vi "BuildUpdateQuery.vi"(8 "error in (no error)":errorcluster, 10 "QueryBuilderData":T1) -> (0 "error out":errorcluster, 2 "Query":string)   [LabVIEW 2022 SP3]
uses:
  DataTypes/QuiryBuilderData--Cluster.ctl
  <vilib>/Utility/error.llb/Trim Whitespace One-Sided.vi
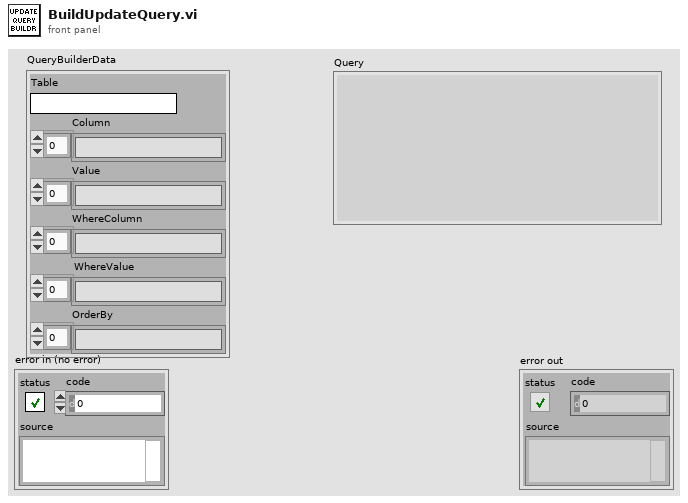
[diagram p1: front panel]
types:
  T1 = typedef "QuiryBuilderData--Cluster.ctl" = cluster{"Table":string, "Column":string[], "Value":string[], "WhereColumn":string[], "WhereValue":string[], "OrderBy":string[]}
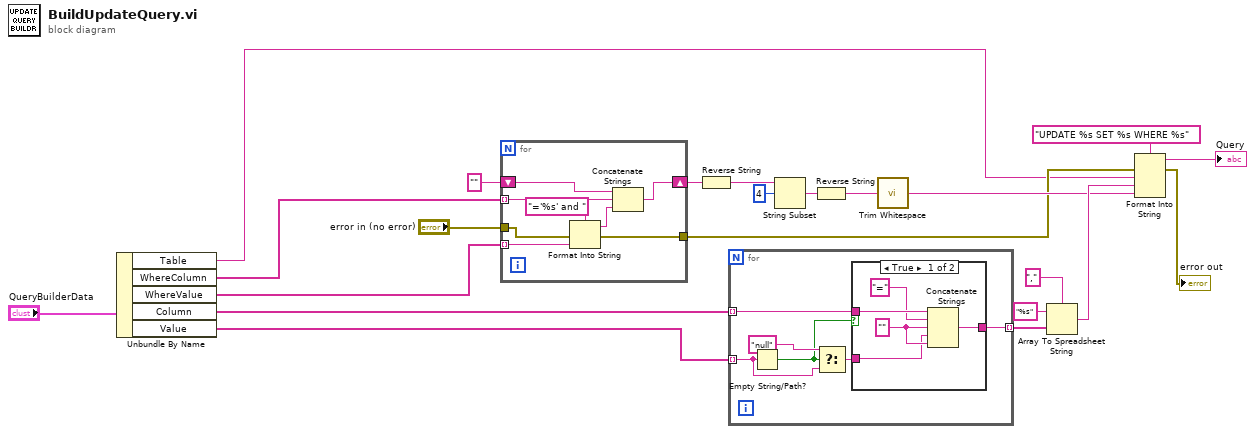
[diagram p0: block diagram]
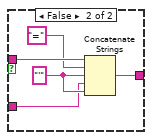
[diagram p2: hidden frame]
diagram:
  n1 = Unbundle By Name("QueryBuilderData") -> ("Table"=w2:string, "WhereColumn"=w3:string[], "WhereValue"=w4:string[], "Column"=w6:string[], "Value"=w5:string[])
  n2 = for {
    tunnel: w3 -> [w30] mode=indexing
    shift-right: [w29] -> w16
    shift-left: "" -> [w28]
    tunnel: w4 -> [w25] mode=indexing
    tunnel: "error in (no error)" -> [w24]
    tunnel: [w23] -> w9
    n3 = Format Into String(format string="='%s' and " ("string"), error in=w24, w25) -> (resulting string=w26:string, error out=w23:errorcluster)  [unwired: 1 in]
    n4 = Concatenate Strings(w28, w30, w26) -> (w29:string)
  }
  n5 = Reverse String(1:w16) -> (0:w14:string)
  n6 = for {
    tunnel: w6 -> [w36] mode=indexing
    tunnel: w5 -> [w32] mode=indexing
    tunnel: [w35] -> w21 mode=indexing
    n7 = Empty String/Path?(string/path=w32) -> (empty?=w31:bool)
    n8 = Select(t="null" ("string"), s=w31, f=w32) -> (s? t:f=w34:string)
    n9 = case shown="True" w31 {
      tunnel: w36 -> [w41 w46]
      tunnel: [w38 w43] -> w35
      tunnel: w34 -> [w37 w42]
      frame True {
        w39 = "" ("string")
        n10 = Concatenate Strings(w41, "=" ("string"), w39, w37, w39) -> (w38:string)
      }
      frame False {
        w44 = "'" ("string")
        n11 = Concatenate Strings(w46, "=" ("string"), w44, w42, w44) -> (w43:string)
      }
    }
  }
  n12 = String Subset(string=w14, offset (0)=4) -> (substring=w13:string)  [unwired: 1 in]
  n13 = Reverse String(1:w13) -> (0:w11:string)
  n14 = call <vilib>:"Trim Whitespace.vi"("string"=w11) -> ("trimmed string"=w12:string)  [unwired: 1 in]
  n15 = Array To Spreadsheet String(delimiter (Tab)=",", array=w21, 3:"%s" ("format string")) -> (spreadsheet string=w18:string)
  n16 = Format Into String(format string="UPDATE %s SET %s WHERE %s", error in=w9, w2, w18, w12) -> (resulting string=→"Query":string, error out=→"error out":errorcluster)  [unwired: 1 in]
